vi "Read CAN Data.vi"(8 "error in (no error)":errorcluster, 11 "OrionBMS in":refnum<class "Orion_BMS.lvclass">) -> (0 "error out":errorcluster, 2 "CAN Data":T1, 3 "OrionBMS out":refnum<class "Orion_BMS.lvclass">)   [LabVIEW 2017, in "Orion_BMS.lvclass"]
uses:
  Orion_BMS.lvclass
  TypeDef_CANData.ctl
  TypeDef_BmsStatus.ctl
  Orion_BMS.lvclass/Orion_BMS.ctl
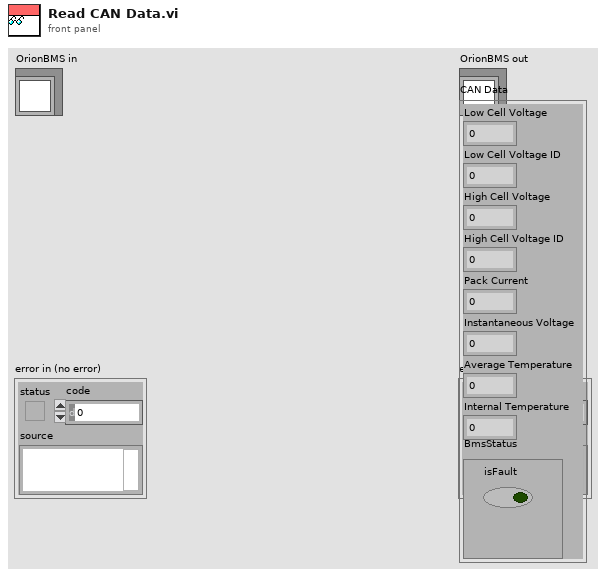
[diagram p1: front panel]
types:
  T1 = typedef "TypeDef_CANData.ctl" = cluster{"Low Cell Voltage":dbl, "Low Cell Voltage ID":dbl, "High Cell Voltage":dbl, "High Cell Voltage ID":dbl, "Pack Current":dbl, "Instantaneous Voltage":dbl, "Average Temperature":dbl, "Internal Temperature":dbl, "BmsStatus":T2}
  T2 = typedef "TypeDef_BmsStatus.ctl" = cluster{"isFault":bool}
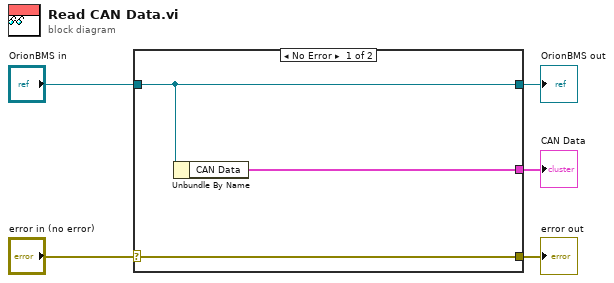
[diagram p0: block diagram]
diagram:
  n1 = case shown="No Error" "error in (no error)" {
    selector: "error in (no error)" -> [w8 w9]
    tunnel: [w8 w9] -> w4
    tunnel: [w7 w10] -> w2
    tunnel: "OrionBMS in" -> [w7 w10]
    tunnel: [w6 _] -> w1
    frame No Error {
      n2 = Unbundle By Name(w7) -> ("CAN Data"=w6:T1)
    }
    frame Error {
    }
  }
  "error out" <- w4
  "OrionBMS out" <- w2
  "CAN Data" <- w1
